vi "Send Command.vi"(4 "message attributes":T1, 6 "timeout (-1 ms)":i32=-1, 8 "error in (no error)":errorcluster, 9 "message value":string, 10 "message name":string, 11 "VeriStand Comm in":refnum<class "VeriStand Comm.lvclass">) -> (0 "error out":errorcluster, 3 "VeriStand Comm out":refnum<class "VeriStand Comm.lvclass">)   [LabVIEW 2018, in "NI VeriStand Addon Network Comm.lvlib" / "VeriStand Comm.lvclass"]
uses:
  VeriStand Comm.lvclass
  <vilib>/NI/Tools/Keyed Array/KeyedArray.ctl
  VeriStand Comm.lvclass/VeriStand Comm.ctl
  <vilib>/NI/AMC/Create Single Message.vi
  <vilib>/NI/AMC/Update Message Routing Info.vi
  <vilib>/NI/AMC/Send Message.vi
  <vilib>/NI/AMC/AMC.lvlib
  <vilib>/NI/Tools/Keyed Array/Tools_KeyedArray.lvlib
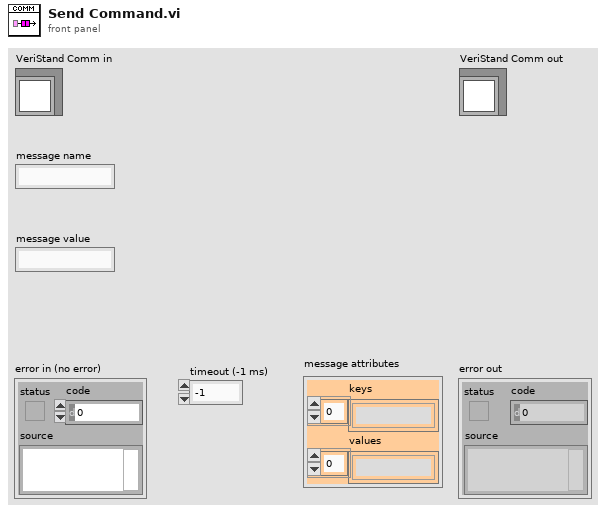
[diagram p1: front panel]
types:
  T1 = typedef "Tools_KeyedArray.lvlib/KeyedArray.ctl" = cluster{"keys":string[], "values":string[]}
  T2 = typedef "AMC.lvlib/Message Queue.ctl" = refnum<queue>
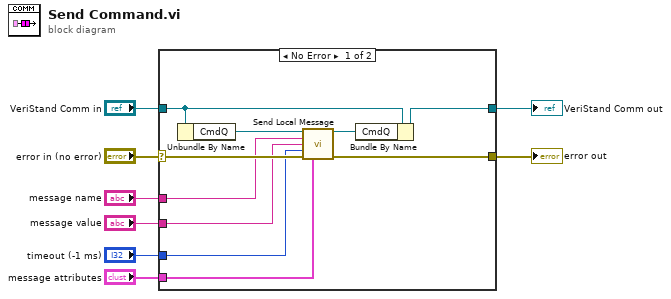
[diagram p0: block diagram]
diagram:
  n1 = case shown="No Error" "error in (no error)" {
    selector: "error in (no error)" -> [w17 w20]
    tunnel: [w18 w20] -> w7
    tunnel: [w10 w19] -> w5
    tunnel: "VeriStand Comm in" -> [w11 w19]
    tunnel: "message value" -> [w16 _]
    tunnel: "timeout (-1 ms)" -> [w15 _]
    tunnel: "message name" -> [w13 _]
    tunnel: "message attributes" -> [w9 _]
    frame No Error {
      n2 = Unbundle By Name(w11) -> ("CmdQ"=w14:T2)
      n3 = call <vilib>:"Send Local Message.vi"("message queue in"=w14, "message name"=w13, "message value"=w16, "timeout (-1 ms)"=w15, "error in"=w17, "message attributes"=w9) -> ("message queue out"=w12:T2, "error out"=w18:errorcluster)  [unwired: 7 in, 1 out]
      n4 = Bundle By Name(cluster=w11, "CmdQ"=w12) -> (w10:refnum<class "VeriStand Comm.lvclass">)
    }
    frame Error {
    }
  }
  "error out" <- w7
  "VeriStand Comm out" <- w5
